vi "VHM-getDataSet.vi"(8 "error in (no error)":errorcluster, 11 "VHM-VNA_Hardware_Manager in":refnum<class "VHM-VNA_Hardware_Manager.lvclass">) -> (0 "error out":errorcluster, 2 "VNA data":T2, 3 "VHM-VNA_Hardware_Manager out":refnum<class "VHM-VNA_Hardware_Manager.lvclass">)   [LabVIEW 2020, in "VHM-VNA_Hardware_Manager.lvlib" / "VHM-VNA_Hardware_Manager.lvclass"]
uses:
  VHM-VNA_Hardware_Manager.lvclass
  classes/vna-drivers/liteVNA/VD-VNA_data.ctl
  classes/vna-drivers/liteVNA/VD-data_read_status.ctl
  VHM-VNA_Hardware_Manager.lvclass/VHM-VNA_Hardware_Manager.ctl
  VHMI-VNA_Hardware_manager_Interface Messages/VHMI-recieveData Msg/VHMI-recieveData Msg.lvclass/VHMI-recieveData Msg.ctl
  <vilib>/ActorFramework/Message Enqueuer/Message Enqueuer.lvclass/Message Enqueuer.ctl
  <vilib>/ActorFramework/Message Enqueuer/Enqueue.vi
  VHMI-VNA_Hardware_manager_Interface Messages/VHMI-recieveData Msg/VHMI-recieveData Msg.lvclass
  C:/Program Files (x86)/National Instruments/LabVIEW 2020/vi.lib/ActorFramework/Message/Message.lvclass
  <vilib>/ActorFramework/Message Priority Queue/Priority Enqueue.vi
  classes/vna-drivers/liteVNA/VD-LV-LiteVNA.lvclass
panel:
  out "Valid Data?":bool
  out "data status":T1
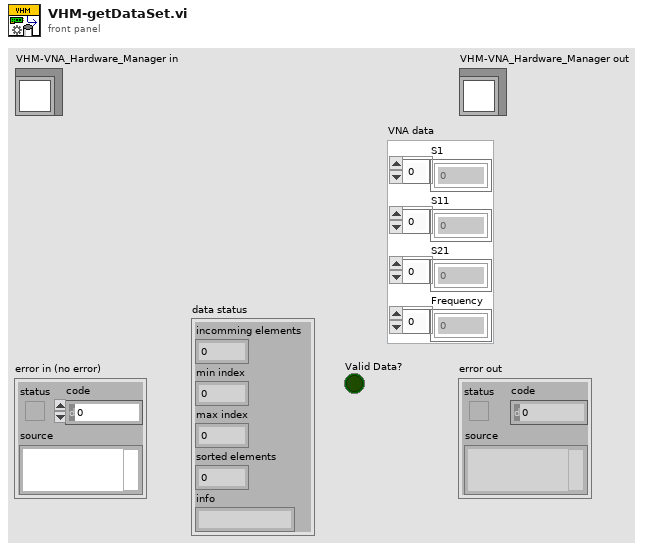
[diagram p1: front panel]
types:
  T1 = typedef "VD-LV-LiteVNA.lvclass/VD-data_read_status.ctl" = cluster{"incomming elements":i32, "min index":u16, "max index":u16, "sorted elements":i32, "info":string}
  T2 = typedef "VD-LV-LiteVNA.lvclass/VD-VNA_data.ctl" = cluster{"S1":cdb[], "S11":cdb[], "S21":cdb[], "Frequency":u64[]}
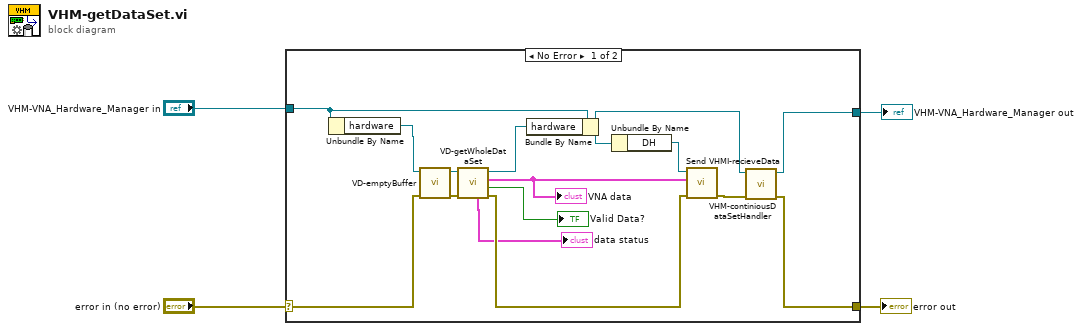
[diagram p0: block diagram]
diagram:
  n1 = case shown="No Error" "error in (no error)" {
    selector: "error in (no error)" -> [w18 w21]
    tunnel: [w7 w21] -> w3
    tunnel: [w5 w20] -> w1
    tunnel: "VHM-VNA_Hardware_Manager in" -> [w19 w20]
    frame No Error {
      n2 = Unbundle By Name(w19) -> ("hardware"=w17:refnum<class "VD-LV-LiteVNA.lvclass">)
      n3 = call-dynamic "VD-emptyBuffer.vi"("error in (no error)"=w18, "VD-LV-LiteVNA in"=w17) -> ("error out"=w15:errorcluster, "VD-LV-LiteVNA out"=w14:refnum<class "VD-LV-LiteVNA.lvclass">)  [unwired: 5 in, 3 out]
      n4 = call-dynamic "VD-getWholeDataSet.vi"("error in (no error)"=w15, "VD-LV-LiteVNA in"=w14) -> ("error out"=w10:errorcluster, "Valid Data?"=→"Valid Data?":bool, "VNA data"=w12:T2, "VD-LV-LiteVNA out"=w13:refnum<class "VD-LV-LiteVNA.lvclass">, "data status"=→"data status":T1)  [unwired: 5 in]
      "VNA data" <- w12
      n5 = Bundle By Name(cluster=w19, "hardware"=w13) -> (w6:refnum<class "VHM-VNA_Hardware_Manager.lvclass">)
      n6 = Unbundle By Name(w6) -> ("DH"=w16:refnum<class "Message Enqueuer.lvclass">)
      n7 = call "Send VHMI-recieveData.vi"("error in (no error)"=w10, "VNA data"=w12, "Message Enqueuer"=w16) -> ("error out"=w8:errorcluster)  [unwired: 7 in, 1 out]
      n8 = call "VHM-continiousDataSetHandler.vi"("error in (no error)"=w8, "VHM-VNA_Hardware_Manager in"=w6) -> ("error out"=w7:errorcluster, "VHM-VNA_Hardware_Manager out"=w5:refnum<class "VHM-VNA_Hardware_Manager.lvclass">)  [unwired: 8 in]
    }
    frame Error {
    }
  }
  "error out" <- w3
  "VHM-VNA_Hardware_Manager out" <- w1
